vi "is StateMachineObject.vi"(8 "error in (no error)":errorcluster, 11 "SMO":refnum<class "SMO.lvclass">) -> (0 "error out":errorcluster, 2 "is SMO?":bool, 3 "SMO out":refnum<class "SMO.lvclass">)   [LabVIEW 2013, in "SMO.lvclass"]
uses:
  SMO.lvclass
  SMO.lvclass/SMO.ctl
panel:
  # "For instructions on how to use the JKI State Machine Objects, examples and video tutorials, visit:\nhttp://jki.net/state-machine-objects/\n\nJKI State Machine Objects™\nhttp://jki.net/state-machine-objects/\nCopyright (C) 2005-2015, JKI <info@jki.net>\nALL RIGHTS RESERVED"
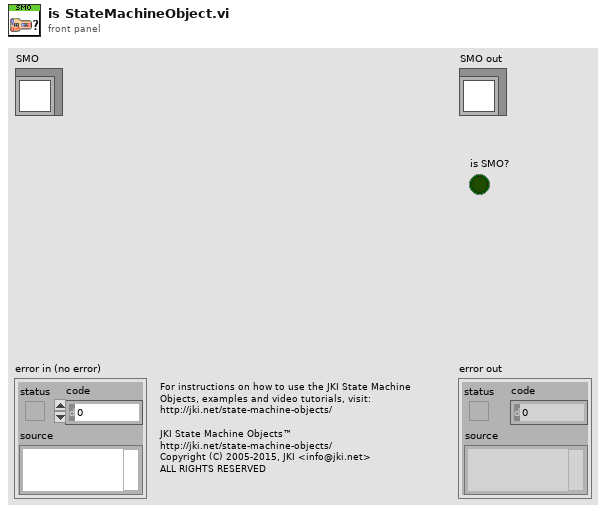
[diagram p1: front panel]
types:
  T1 = typedef "SMO.lvclass/PrivateData--Ref.ctl" = refnum<data-value>
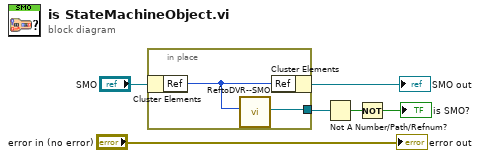
[diagram p0: block diagram]
diagram:
  n1 = in-place {
    in-place-border: [w7] -> w4
    n2 = in-place-cluster #1("SMO") -> ("Ref"=w8:u32)
    n3 = call "ReftoDVR--SMO.vi"("Ref"=w8) -> ("Ref"=w7:T1)  [unwired: 10 in]
    n4 = in-place-cluster #1("Ref"=w8) -> (→"SMO out":refnum<class "SMO.lvclass">)
  }
  n5 = Not A Number/Path/Refnum?(number/path/refnum=w4) -> (NaN/Path/Refnum?=w3:bool)
  n6 = Not(x=w3) -> (.not. x?=→"is SMO?":bool)
  "error out" <- "error in (no error)"
